vi "ReadPUIDs.vi"(8 "error in (no error)":errorcluster) -> (0 "error out":errorcluster, 1 "JSON":string, 2 "PUIDs":string[](array[string]))   [LabVIEW 2015, in "PersonnelRestApi.lvlib"]
uses:
  PersonnelRestApi.lvlib
  TypeDef/GetPersonnelCommands.ctl
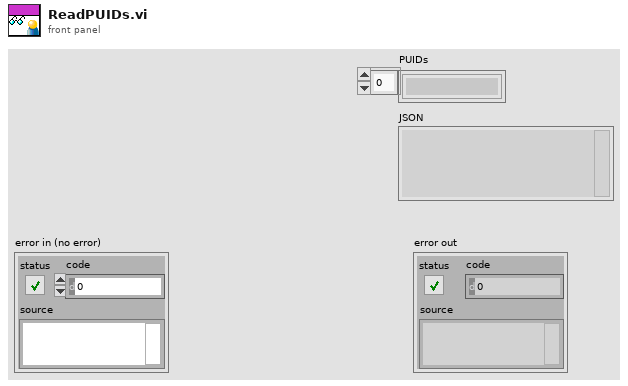
[diagram p1: front panel]
types:
  T1 = typedef "PersonnelRestApi.lvlib/GetPersonnelCommands.ctl" = enum16{"ReadPersonnel", "ReadName", "ReadRole", "ReadRequests", "ReadPUIDs", "ReadAllPersonnel"}
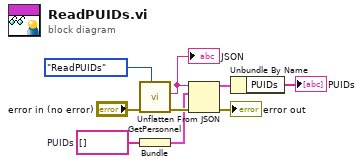
[diagram p0: block diagram]
diagram:
  w4 = string[] []  # PUIDs
  n1 = call "GetPersonnel.vi"("Room Commands"=GetPersonnelCommands."ReadPUIDs", "error in (no error)"="error in (no error)") -> ("error out"=w6:errorcluster, "JSON"=w7:string)  [unwired: 8 in]
  "JSON" <- w7
  n2 = Bundle("PUIDs"=w4) -> (w3:cluster{"PUIDs":string[]})  [unwired: 1 in]
  n3 = Unflatten From JSON(JSON string=w7, type and defaults=w3, error in (no error)=w6) -> (value=w2:cluster{"PUIDs":string[]}, error out=→"error out":errorcluster)  [unwired: 4 in]
  n4 = Unbundle By Name(w2) -> ("PUIDs"=→"PUIDs":string[])
